vi "Init Step.vi"(0 "reference in":refnum<class "Stand.lvclass">, 1 "init":bool, 11 "error in (no error)":errorcluster) -> (4 "reference out":refnum<class "Stand.lvclass">, 6 "done":bool, 15 "error out":errorcluster)   [LabVIEW 2019, in "Stand.lvclass"]
uses:
  Stand.lvclass
  C:/Users/ANENKOV_V1/Desktop/src/Device_class/Device.lvclass
  FPGA/TypeDef/DO index.ctl
  Valve DIR.ctl
  Device_class/Device.lvclass/Device.ctl
  Stand.lvclass/Stand.ctl
  TypeDef/Active Motor.ctl
  TypeDef/Motor N.ctl
  Valve_2DO_2DI_class/CMD.ctl
  NeedleValve_class/Cmd.ctl
  DoValve.vi
  DoValve.vi/e7d2c9dc-ba67-4685-b926-bcce34aa2778.vi
  DoValve.vi/628819af-fd07-4303-9780-3ddd467101db.vi
  Const All Valve.vi
  FPGA_API_class/FPGA API.lvclass
  Device_class/Device.lvclass
  PM_Group_class/PM_Group.lvclass
  Valve_2DO_2DI_class/Valve_2DO_2DI.lvclass
  NeedleValve_class/NeedleValve.lvclass
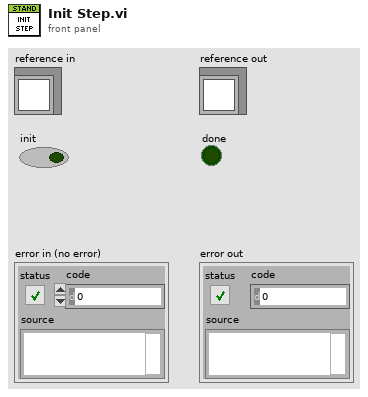
[diagram p1: front panel]
types:
  T1 = typedef "Valve DIR.ctl" = enum16{"Air Valves: Open (DUT Filling)", "Air Valves: Open (Chamber Filling)", "Air Valves: Open (Pump Pressure DUT)", "Air Valves: Open (Pump Pressure Chamber)", "Air Valves: Open (Haskel Pressure DUT)", "Air Valves: Open (Haskel Pressure Chamber)", "Air Valves: Open (Slow Release DUT)", "Air Valves: Open (Slow Release Chamber)", "Air Valves: Open (Fast Release DUT)", "Air Valves: Open (Fast Release Chamber)", "Air Valves: Open (Emergency Release DUT and Chamber)", "Air Valves: Leak Hi (Chamber)", "Air Valves: Leak Hi (DUT)", "Air Valves: Backpressure (Chamber)", "Air Valves: Backpressure (DUT)", "Air Valves: Fully Closed", "Air Valves: Open 33.7"}
  T2 = typedef "DO index.ctl" = u8
  T3 = typedef "Direction.ctl" = enum8{"DUT", "Chamber"}
  T4 = typedef "NeedleValve.lvclass/Cmd.ctl" = enum16{"Open", "Close", "Stop"}
  T5 = typedef "Active Motor.ctl" = cluster{"Active":bool, "MotorN":T6}
  T6 = typedef "Motor N.ctl" = enum16{"M12", "M21", "M24"}
  T7 = typedef "Valve_2DO_2DI.lvclass/CMD.ctl" = enum16{"Open", "Close"}
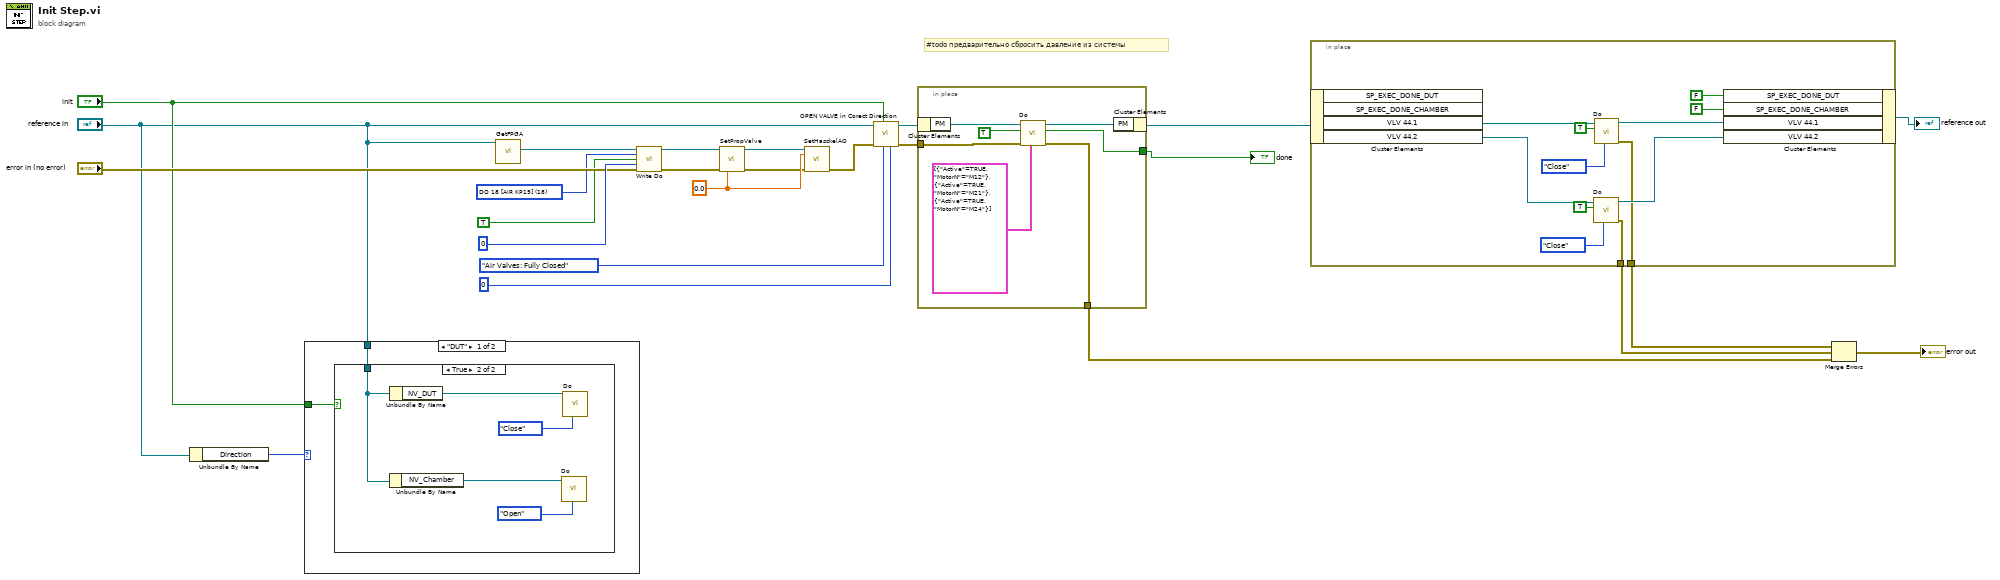
[diagram p0: block diagram]
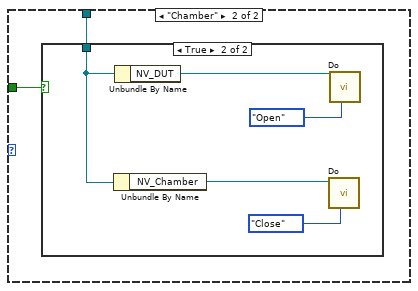
[diagram p3: hidden frame]
diagram:
  w19 = 0.0 ("AO 1")
  w6 = T2 18 items=["DO 0 [KP1] [M12]", "DO 1 [ON KP2] [M21]", "DO 2 [ON KP3] [M24]", "DO 3 [WATER Y18.1 [DO3]]", "DO 4 [WATER Y18.2 [DO4]]", "DO 5 [KP6 Y29.1 33.7]", "DO 6 [KP7 Y29.2 33.8]", "DO 7 [KP8 Y29.3 33.9]", "DO 8 [KP9 Y29.4  33.12]", "DO 9 [KP10 Y29.5 33.1]", "DO 10 [KP11 Y29.6 33.2]", "DO 11 [KP12 Y29.7  33.13]", "DO 12 [KP13 Y29.8  33.11]", "DO 13 [KP14 Y29.9 33.10]", "DO 14 [KP15 Y29.10  33.6]", "DO 15 [KP16 Y29.11  33.5]", "DO 16 [KP17 Y29.12  33.4]", "DO 17 [KP18 Y29.13 33.3]", "DO 18 [AIR KP19]", "DO 19 [STEP DRIVE EN KP20]", "DO 20 [KP21 Y44.1 OPEN]", "DO 21 [ KP22 Y44.1 CLOSE]", "DO 22 [ KP23 Y44.2 OPEN]", "DO 23", "DO 24 [STEP DRIVE 1]", "DO 25 [STEP DRIVE 2]"] ("#DO")
  # "#todo предварительно сбросить давление из системы"
  n1 = Unbundle By Name("reference in") -> ("Direction"=w4:T3)
  n2 = case shown="\"DUT\"" w4 {
    tunnel: "reference in" -> [w27 w34]
    tunnel: "init" -> [w26 w33]
    frame "DUT" {
      n3 = case shown="True" w26 {
        tunnel: w27 -> [_ w32]
        frame False {
        }
        frame True {
          n4 = Unbundle By Name(w32) -> ("NV_Chamber"=w28:refnum<class "NeedleValve.lvclass">)
          n5 = Unbundle By Name(w32) -> ("NV_DUT"=w30:refnum<class "NeedleValve.lvclass">)
          n6 = call "Do.vi"("Cmd"=Cmd."Open", "NeedleValve in"=w28) -> ()  [unwired: 8 in, 2 out]
          n7 = call "Do.vi"("Cmd"=Cmd."Close", "NeedleValve in"=w30) -> ()  [unwired: 8 in, 2 out]
        }
      }
    }
    frame "Chamber" {
      n8 = case shown="True" w33 {
        tunnel: w34 -> [_ w39]
        frame False {
        }
        frame True {
          n9 = Unbundle By Name(w39) -> ("NV_Chamber"=w35:refnum<class "NeedleValve.lvclass">)
          n10 = Unbundle By Name(w39) -> ("NV_DUT"=w37:refnum<class "NeedleValve.lvclass">)
          n11 = call "Do.vi"("Cmd"=Cmd."Close", "NeedleValve in"=w35) -> ()  [unwired: 8 in, 2 out]
          n12 = call "Do.vi"("Cmd"=Cmd."Open", "NeedleValve in"=w37) -> ()  [unwired: 8 in, 2 out]
        }
      }
    }
  }
  n13 = call "GetFPGA.vi"("Device in"="reference in") -> ("FPGA API.lvclass"=w7:refnum<class "FPGA API.lvclass">)  [unwired: 10 in]
  n14 = call-dynamic "Write Do.vi"("FPGA API in"=w7, "#DO"=w6, "value"=TRUE, "Time uSec"=u32 0, "error in (no error)"="error in (no error)") -> ("FPGA API out"=w14:refnum<class "FPGA API.lvclass">, "error out"=w15:errorcluster)  [unwired: 9 in]
  n15 = call-dynamic "SetPropValve.vi"("FPGA API in"=w14, "error in (no error)"=w15, "AO 1"=w19) -> ("FPGA API out"=w16:refnum<class "FPGA API.lvclass">, "error out"=w17:errorcluster)  [unwired: 11 in]
  n16 = call-dynamic "SetHasckelAO.vi"("FPGA API in"=w16, "Haskel in"=w19, "error in (no error)"=w17) -> ("error out"=w18:errorcluster)  [unwired: 11 in, 1 out]
  n17 = call "OPEN VALVE in Corect Direction.vi"("time after close"=u32 0, "Valve DIR"=Valve_DIR."Air Valves: Fully Closed", "changed or first call?"="init", "error in (no error)"=w18, "Stand in"="reference in") -> ("error out"=w11:errorcluster, "Stand out"=w10:refnum<class "Stand.lvclass">)  [unwired: 4 in, 1 out]
  n18 = in-place {
    in-place-border: w11 -> [w45]
    in-place-border: [w43] -> w24
    in-place-border: [w40] -> w20
    n19 = in-place-cluster #1(w10) -> ("PM"=w46:refnum<class "PM_Group.lvclass">)
    n20 = call "Do.vi"("Data"=T5[] [{"Active"=TRUE, "MotorN"=enum."M12"}, {"Active"=TRUE, "MotorN"=enum."M21"}, {"Active"=TRUE, "MotorN"=enum."M24"}] ("Array"), "error in (no error)"=w45, "Do"=TRUE, "PM_Group in"=w46) -> ("error out"=w43:errorcluster, "Done"=w40:bool, "PM_Group out"=w44:refnum<class "PM_Group.lvclass">)  [unwired: 5 in]
    n21 = in-place-cluster #1("PM"=w44) -> (w3:refnum<class "Stand.lvclass">)
  }
  "done" <- w20
  n22 = in-place {
    in-place-border: [w50] -> w22
    in-place-border: [w49] -> w23
    n23 = in-place-cluster #2(w3) -> ("VLV 44.1"=w58:refnum<class "Valve_2DO_2DI.lvclass">, "VLV 44.2"=w52:refnum<class "Valve_2DO_2DI.lvclass">)  [unwired: 2 out]
    n24 = call "Do.vi"("CMD"=CMD."Close", "Do"=TRUE, "Valve_2DO_2DI in"=w52) -> ("error out"=w50:errorcluster, "Valve_2DO_2DI out"=w51:refnum<class "Valve_2DO_2DI.lvclass">)  [unwired: 6 in, 1 out]
    n25 = call "Do.vi"("CMD"=CMD."Close", "Do"=TRUE, "Valve_2DO_2DI in"=w58) -> ("error out"=w49:errorcluster, "Valve_2DO_2DI out"=w57:refnum<class "Valve_2DO_2DI.lvclass">)  [unwired: 6 in, 1 out]
    n26 = in-place-cluster #2("SP_EXEC_DONE_DUT"=FALSE ("Data.STS.SP_EXEC_DONE_DUT"), "SP_EXEC_DONE_CHAMBER"=FALSE ("Data.STS.SP_EXEC_DONE_CHAMBER"), "VLV 44.1"=w57, "VLV 44.2"=w51) -> (→"reference out":refnum<class "Stand.lvclass">)
  }
  n27 = Merge Errors(w23, w22, w24) -> (→"error out":errorcluster)
